vi "Get Number of Active Axes.vi"() -> (0 "error out":errorcluster, 3 "value":i32)   [LabVIEW 2019, in "ESP301.lvlib"]
uses:
  ESP301.lvlib
  <vilib>/Utility/config.llb/Read Key (I32).vi
  <vilib>/Utility/config.llb/NI_LVConfig.lvlib
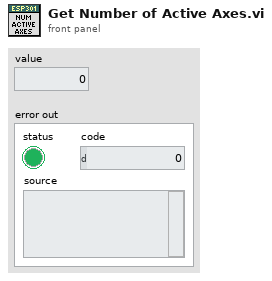
[diagram p1: front panel]
types:
  T1 = typedef "NI_LVConfig.lvlib/Config Data RefNum.ctl" = refnum<k1>
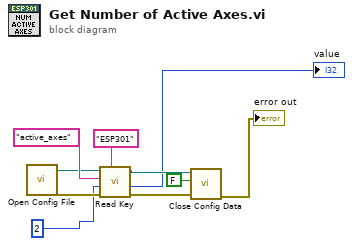
[diagram p0: block diagram]
diagram:
  n1 = call "Open Config File.vi"() -> ("error out"=w8:errorcluster, "Refnum out"=w7:T1)  [unwired: 10 in]
  n2 = call-poly <vilib>:"Read Key.vi"("section"="ESP301", "error in (no error)"=w8, "default value"=2, "key"="active_axes", "refnum"=w7) -> ("error out"=w4:errorcluster, "value"=→"value":i32, "refnum out"=w5:T1)  [unwired: 3 in, 1 out]
  n3 = call <vilib>:"Close Config Data.vi"("error in (no error)"=w4, "write file if changed (T)"=FALSE, "refnum"=w5) -> ("error out"=→"error out":errorcluster)  [unwired: 7 in, 1 out]
